vi "Access Handle.vi"(8 "error in (no error)":errorcluster, 11 "Buffer":refnum<class "Buffer.lvclass">) -> (0 "error out":errorcluster, 3 "Handle":refnum<data-value>)   [LabVIEW 2020, in "Buffer.lvclass"]
uses:
  Buffer.lvclass
  Buffer.lvclass/Buffer.ctl
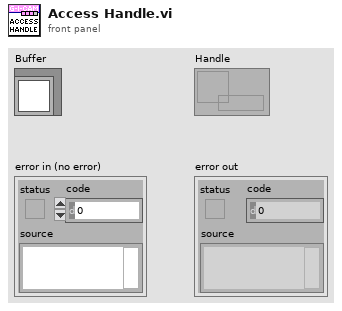
[diagram p1: front panel]
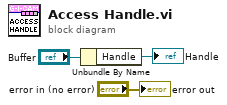
[diagram p0: block diagram]
diagram:
  n1 = Unbundle By Name("Buffer") -> ("Handle"=→"Handle":refnum<data-value>)
  "error out" <- "error in (no error)"
